vi "SubnetScanIPs.vi"() -> ()   [LabVIEW 2011]
doc: "This VI will scan all addresses in a simple subnet, to aid in finding \"lost\" devices."
panel:
  in  "Stop Button":bool
  out "Found devices":string[](array[string])
  in  "timeout ms":i32=100
  in  "Port to test":u16=80
  in  "Subnet to test":string="69.162.55"
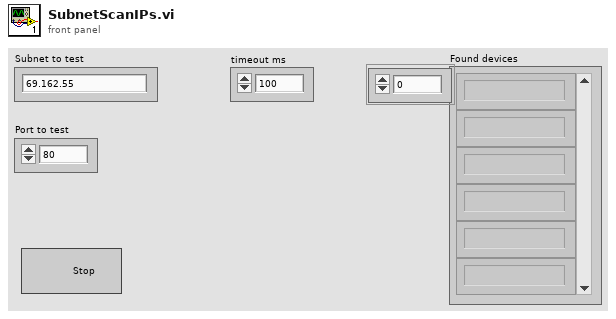
[diagram p1: front panel]
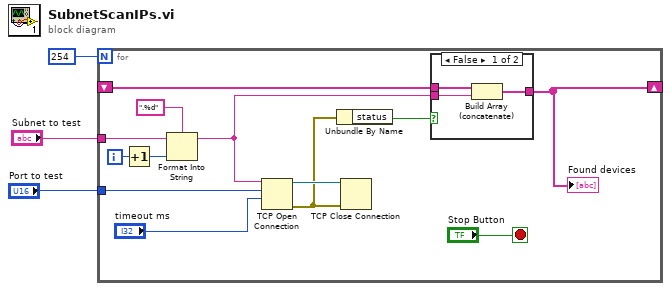
[diagram p0: block diagram]
diagram:
  n1 = for {
    N: 254 -> [_]
    tunnel: "Port to test" -> [w15]
    tunnel: "Subnet to test" -> [w14]
    shift-right: [w4] -> _
    shift-left: _ -> [w8]
    i -> [w13]
    stop <- "Stop Button" stop-if-true
    n2 = Increment(x=w13) -> (x+1=w12:i32)
    n3 = Format Into String(format string=".%d", initial string=w14, w12) -> (resulting string=w5:string)  [unwired: 1 in, 1 out]
    n4 = TCP Open Connection(address=w5, remote port or service name=w15, timeout ms (60000)="timeout ms") -> (connection ID=w16:refnum<k5>, error out=w9:errorcluster)  [unwired: 2 in]
    n5 = Unbundle By Name(w9) -> ("status"=w7:bool)
    n6 = TCP Close Connection(connection ID=w16, error in (no error)=w9) -> ()  [unwired: 1 in, 2 out]
    n7 = case shown="False" w7 {
      tunnel: w5 -> [w17 _]
      tunnel: w8 -> [w19 w20]
      tunnel: [w18 w20] -> w4
      frame False {
        n8 = Build Array (concatenate)(w19, w17) -> (w18:string[])
      }
      frame True {
      }
    }
    "Found devices" <- w4
  }
